vi "WritePAQsample.vi"(8 "error in (no error)":errorcluster, 9 "DAQ-Queue":refnum<queue>, 11 "PAQ IN":T1={"Time Stamp"=timestamp(0 s since 1904-01-01), "TAGs"=[], "status"=[], "data"=[], "Source"="DAQ"} {"data" format="%.2f"; "status" format="%08x"}) -> (0 "error out":errorcluster, 3 "# elements in queue":i32)   [LabVIEW 2020]
doc: "This routine will store one PAQ sample to the data historian.\nThe Array of TAGs is stored into a Queu to minimize load on DAQ code\n\nIf the TAG does not exist: then it will be created.\nThe time of calling this routine is utilized as measurement time.\n\n- Medium speed acquisition (around 6 s/min up to 10 s/sec)\n - Continuous acquisition\n - Usual fixed acquisition speed\n - One timestamp per sample of multiple channels\n - All channels sampled simultaneous\n - Usual non-deterministic (not real time)\n - Typical application field: DCS or MES systems"
uses:
  controls/typedef_PAQsample.ctl
  controls/typedef-DAQ-datagram.ctl
  controls/typedef-Qtype.ctl
panel:
  # "Write Continuous Perioc data to Historian"
  # "Status bit info:"
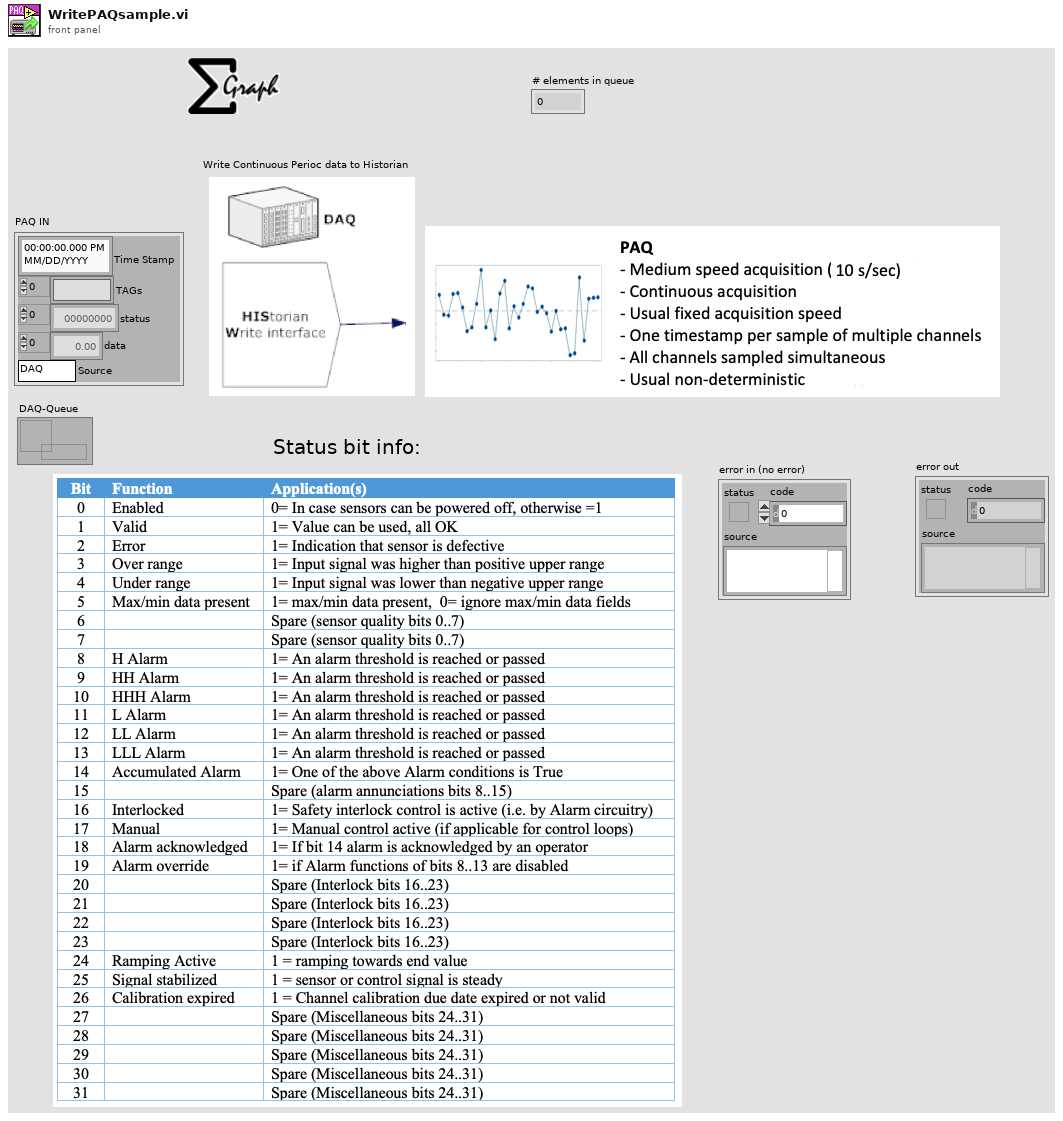
[diagram p1: front panel]
types:
  T1 = typedef "typedef_PAQsample.ctl" = cluster{"Time Stamp":timestamp, "TAGs":string[], "status":u32[], "data":dbl[], "Source":string}
  T2 = typedef "typedef-Qtype.ctl" = enum16{"PAQ", "WAQ", "EAQ", "End-Service"}
  T3 = typedef "typedef-DAQ-datagram.ctl" = cluster{"Time Stamp":timestamp, "Source":string, "Data":variant, "Qtype":T2}
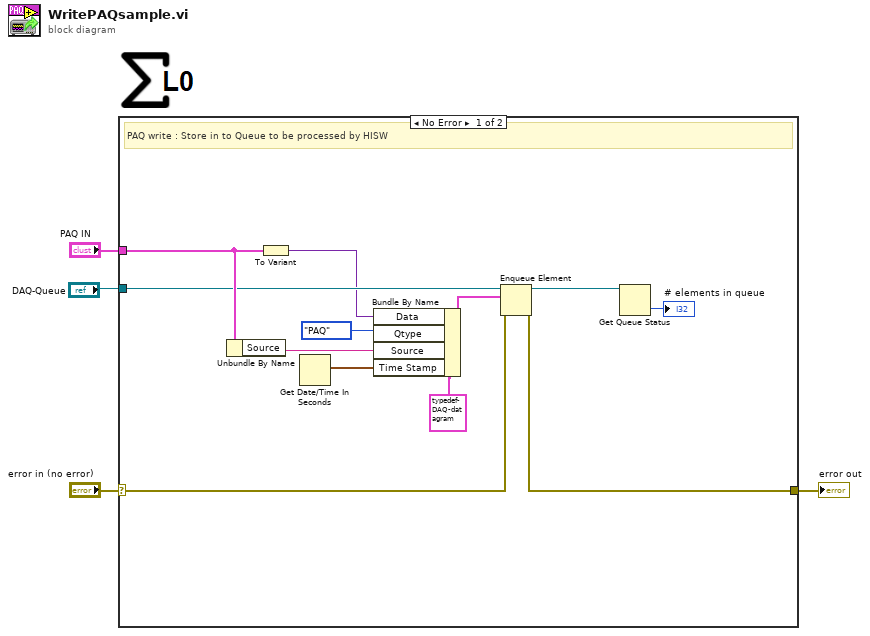
[diagram p0: block diagram]
diagram:
  n1 = case shown="No Error" "error in (no error)" {
    selector: "error in (no error)" -> [w16 w17]
    tunnel: [w14 w17] -> w3
    tunnel: "PAQ IN" -> [w15 _]
    tunnel: "DAQ-Queue" -> [w13 _]
    frame No Error {
      # "PAQ write : Store in to Queue to be processed by HISW"
      n2 = Unbundle By Name(w15) -> ("Source"=w9:string)
      n3 = To Variant(anything=w15) -> (Variant=w6:variant)
      n4 = Get Date/Time In Seconds() -> (seconds since 1Jan1904=w10:timestamp)
      n5 = Bundle By Name(cluster=T3 {"Time Stamp"=timestamp(0 s since 1904-01-01), "Source"="", "Data"=variant, "Qtype"=enum."PAQ"} ("element"), "Data"=w6, "Qtype"=typedef-Qtype."PAQ", "Source"=w9, "Time Stamp"=w10) -> (w7:T3)
      n6 = Enqueue Element(queue=w13, element=w7, error in (no error)=w16) -> (queue out=w12:refnum<queue>, error out=w14:errorcluster)  [unwired: 1 in, 1 out]
      n7 = Get Queue Status(queue=w12) -> (# elements in queue=→"# elements in queue":i32)  [unwired: 2 in, 7 out]
    }
    frame Error {
    }
  }
  "error out" <- w3
